vi "UV_Get_chn stat.vi"(8 "error in (no error)":errorcluster) -> (0 "error out":errorcluster, 2 "chn_actived":bool[](array[boolean]), 3 "VISA resource out":refnum<visa-resource-name>, 5 "Err?":bool)   [LabVIEW 2014]
uses:
  TypeDef/UVLed_func.ctl
  TypeDef/UVLed_channel.ctl
panel:
  in  "VISA resource":refnum<visa-resource-name>="COM5"
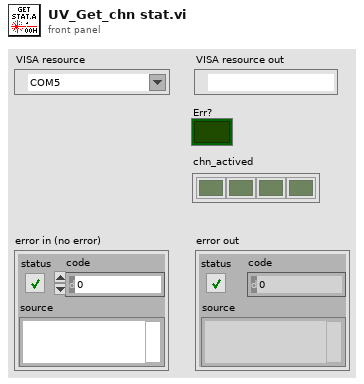
[diagram p1: front panel]
types:
  T1 = typedef "UVLed_channel.ctl" = u16
  T2 = typedef "UVLed_func.ctl" = u16
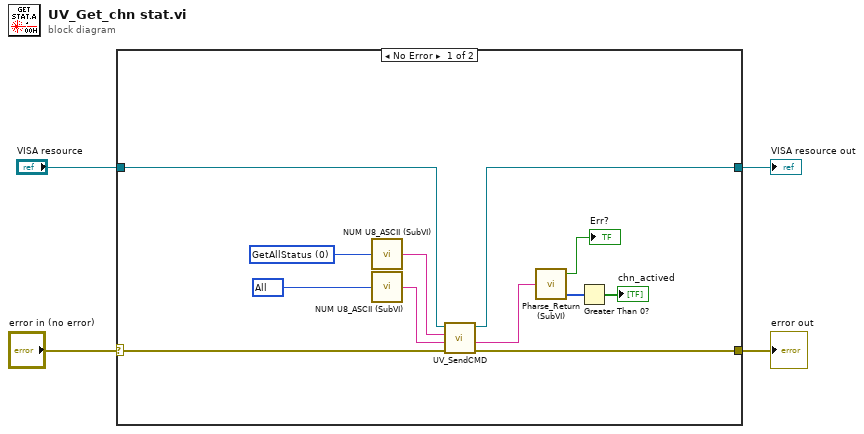
[diagram p0: block diagram]
diagram:
  n1 = case shown="No Error" "error in (no error)" {
    selector: "error in (no error)" -> [w12 w18]
    tunnel: [w10 w18] -> w3
    tunnel: "VISA resource" -> [w13 w17]
    tunnel: [w8 w17] -> w1
    frame No Error {
      w14 = T1 255 items=["All"=255, "CH1"=1, "CH2"=2, "CH3"=3, "CH4"=4] ("CHN")
      w16 = T2 0 items=["GetAllStatus"=0, "LightOn"=2, "LightOff"=4, "AllForceOff"=6, "GetMenuChnPara"=10, "SetMenuChnPara"=12, "GetAutoChnPara"=14, "SetAutoChnPara"=16, "GetMenuTemplate"=18, "SetMenuTemplate"=20, "GetAutoTemplate"=22, "SetAutoTemplate"=24, "GetTemplatePara"=26, "SetTemplatePara"=28, "GetMode"=30, "SetMode"=32, "ChkErr"=240] ("Function")
      n2 = call "NUM U8_ASCII (SubVI).vi"("Numeric"=w16) -> ("String out"=w15:string)
      n3 = call "NUM U8_ASCII (SubVI).vi"("Numeric"=w14) -> ("String out"=w11:string)
      n4 = call "UV_SendCMD.vi"("error in"=w12, "value"=w11, "function"=w15, "VISA resource name"=w13) -> ("error out"=w10:errorcluster, "response"=w9:string, "VISA resource name out"=w8:refnum<visa-resource-name>)  [unwired: 5 in]
      n5 = call "Pharse_Return (SubVI).vi"("buffer in"=w9) -> ("byte array"=w6:u8[], "Err?"=→"Err?":bool)  [unwired: 2 in, 1 out]
      n6 = Greater Than 0?(x=w6) -> (x > 0?=→"chn_actived":bool[])
    }
    frame Error {
    }
  }
  "error out" <- w3
  "VISA resource out" <- w1
